vi "Launch Actor Core.vi"(6 "Debug Alias":string, 8 "error in (no error)":errorcluster, 9 "Open Actor Core front panel?":bool, 10 "Caller's Enqueuer":refnum<class "Message Enqueuer.lvclass">, 11 "Actor in":refnum<class "Actor.lvclass">) -> (0 "error out":errorcluster, 3 "Message Enqueuer out":refnum<class "Message Enqueuer.lvclass">)   [LabVIEW 2020, in "Actor Framework.lvlib" / "Actor.lvclass"]
uses:
  <vilib>/ActorFramework/Actor/Actor.lvclass
  <vilib>/ActorFramework/Message Enqueuer/Message Enqueuer.lvclass
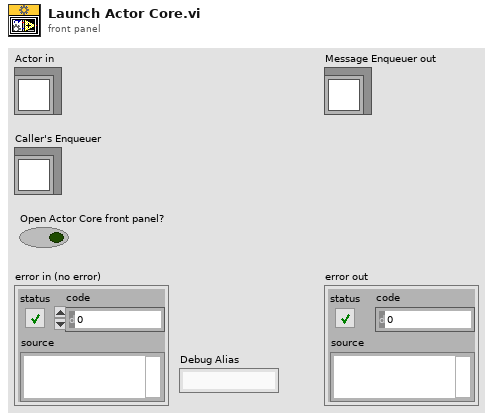
[diagram p1: front panel]
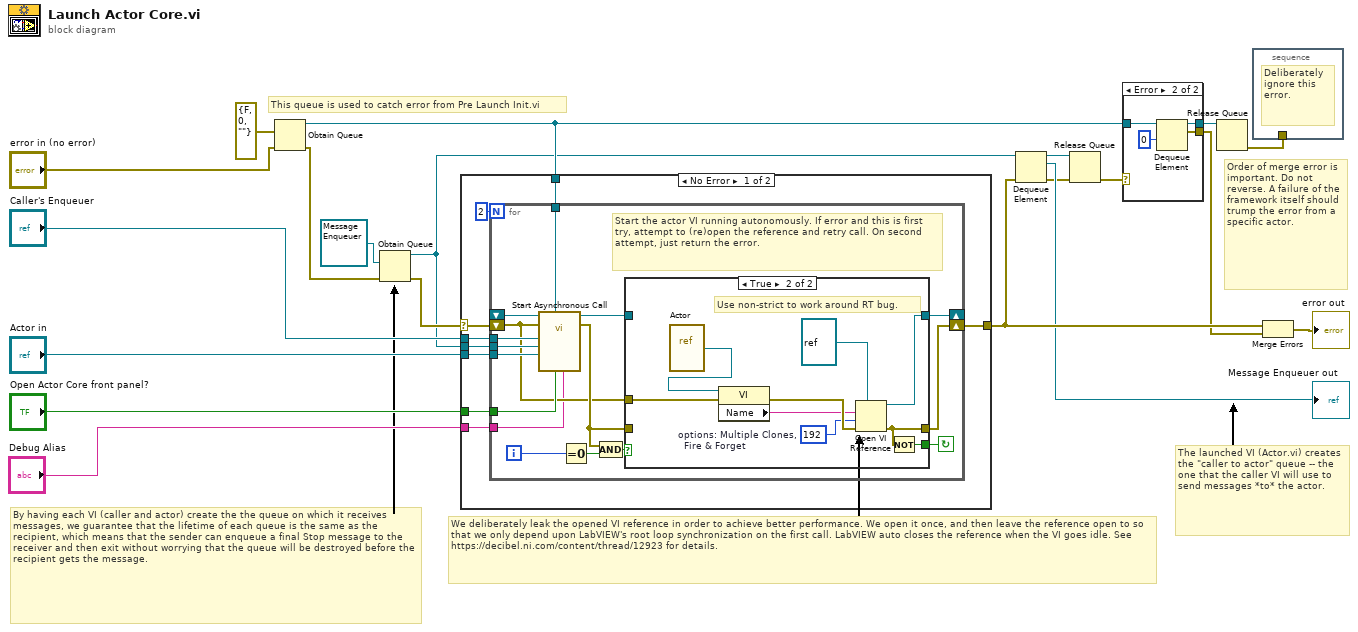
[diagram p0: block diagram]
diagram:
  # "We deliberately leak the opened VI reference in order to achieve better performance. We open it once, and then leave the reference open to so that we only depend upon LabVIEW's root loop synchronization on the first call. LabVIEW auto closes the reference when the VI goes idle. See https://decibel.ni.com/content/thread/12923 for details."
  # "By having each VI (caller and actor) create the the queue on which it receives messages, we guarantee that the lifetime of each queue is the same as the recipient, which means that the sender can enqueue a final Stop message to the receiver and then exit without worrying that the queue will be destroyed before the recipient gets the message."
  # "This queue is used to catch error from Pre Launch Init.vi"
  # "Order of merge error is important. Do not reverse. A failure of the framework itself should trump the error from a specific actor."
  # "The launched VI (Actor.vi) creates the \"caller to actor\" queue -- the one that the caller VI will use to send messages *to* the actor."
  n1 = Obtain Queue(element data type=errorcluster {"status"=FALSE, "code"=0, "source"=""} ("Error"), error in (no error)="error in (no error)") -> (queue out=w12:refnum<queue>, error out=w10:errorcluster)  [unwired: 3 in, 1 out]
  n2 = Obtain Queue(element data type=refnum<class "Message Enqueuer.lvclass"> refnum ("Message Enqueuer"), error in (no error)=w10) -> (queue out=w7:refnum<queue>, error out=w16:errorcluster)  [unwired: 3 in, 1 out]
  n3 = case shown="No Error" w16 {
    selector: w16 -> [w22 w57]
    tunnel: "Actor in" -> [w29 _]
    tunnel: "Caller's Enqueuer" -> [w28 _]
    tunnel: "Open Actor Core front panel?" -> [w27 _]
    tunnel: w7 -> [w26 _]
    tunnel: w12 -> [w25 _]
    tunnel: [w23 w57] -> w17
    tunnel: "Debug Alias" -> [w21 _]
    frame No Error {
      n4 = for {
        N: 2 -> [_]
        tunnel: w29 -> [w45]
        tunnel: w28 -> [w44]
        tunnel: w27 -> [w43]
        tunnel: w26 -> [w42]
        tunnel: w25 -> [w41]
        shift-right: [w40] -> _
        shift-left: _ -> [w39]
        shift-right: [w37] -> w23
        shift-left: w22 -> [w31]
        tunnel: w21 -> [w30]
        i -> [w34]
        stop <- w32 continue-if-true
        # "Start the actor VI running autonomously. If error and this is first try, attempt to (re)open the reference and retry call. On second attempt, just return the error."
        n5 = call-by-ref "Start Asynchronous Call"(reference=w39, error in=w31, "Debug Alias"=w30, "Open Actor Core front panel? (F)"=w43, "error feedback"=w41, "Actor"=w45, "queue of queues"=w42, "Message Enqueuer"=w44) -> (reference out=w38:refnum<vi>, error out=w33:errorcluster)  [unwired: 6 in]
        n6 = Equal To 0?(x=w34) -> (x = 0?=w35:bool)
        n7 = Compound Arithmetic op=AND(w33, w35) -> (w36:bool)
        n8 = case shown="True" w36 {
          tunnel: [w47 w53] -> w40
          tunnel: [w46 w51] -> w37
          tunnel: w38 -> [w47 _]
          tunnel: w33 -> [w46 _]
          tunnel: [_ w52] -> w32
          tunnel: w31 -> [_ w50]
          frame False {
          }
          frame True {
            w54 = 192  # options: Multiple Clones,   Fire & Forget
            # "Use non-strict to work around RT bug."
            n9 = vi-ref <vilib>:"Actor.vi"() -> (w49:refnum<vi>)
            n10 = property class="VI"(reference=w49, error in=w50) -> (error out=w56:errorcluster, "Name"=w55:string)  [unwired: 1 out]
            n11 = Open VI Reference(type specifier VI Refnum (for type only)=refnum<vi> refnum, vi path=w55, options=w54, error in (no error)=w56) -> (vi reference=w53:refnum<vi>, error out=w51:errorcluster)  [unwired: 2 in]
            n12 = Not(x=w51) -> (.not. x?=w52:bool)
          }
        }
      }
    }
    frame Error {
    }
  }
  n13 = Dequeue Element(queue=w7, error in (no error)=w17) -> (queue out=w3:refnum<queue>, element=→"Message Enqueuer out":refnum<class "Message Enqueuer.lvclass">, error out=w4:errorcluster)  [unwired: 1 in, 1 out]
  n14 = Release Queue(queue=w3, error in (no error)=w4) -> (error out=w14:errorcluster)  [unwired: 1 in, 2 out]
  n15 = case shown="Error" w14 {
    selector: w14 -> [w59 _]
    tunnel: w12 -> [w58 w63]
    tunnel: [w59 w61] -> w13
    tunnel: [w58 w60] -> w15
    frame No Error {
    }
    frame Error {
      n16 = Dequeue Element(queue=w63, timeout in ms (-1)=0) -> (queue out=w60:refnum<queue>, element=w61:errorcluster)  [unwired: 1 in, 2 out]
    }
  }
  n17 = Release Queue(queue=w15) -> (error out=w20:errorcluster)  [unwired: 2 in, 2 out]
  n18 = stacked-sequence {
    tunnel: w20 -> [_]
    frame #0 {
      # "Deliberately ignore this error."
    }
  }
  n19 = Merge Errors(w17, w13) -> (→"error out":errorcluster)
